vi "jrg_shellopener2.vi"() -> ()   [LabVIEW 2014]
panel:
  in  "stop":bool
  out "WaveformData":T1
  in  "Waveform index":i32
  out "Waveform Graph":waveform(dbl)(graph)
  out "error out":errorcluster
  # "MSU EFish Lab: EOD Read Display"
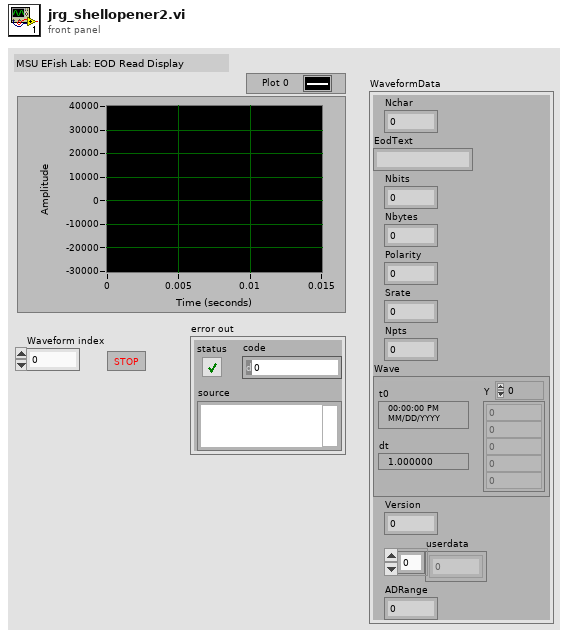
[diagram p1: front panel]
types:
  T1 = cluster{"Nchar":i32, "EodText":string, "Nbits":i32, "Nbytes":i32, "Polarity":i32, "Srate":i32, "Npts":i32, "Wave":waveform(dbl), "Version":i32, "userdata":dbl[], "ADRange":dbl}
  T2 = enum16{"open", "replace", "create", "open or create", "replace or create", "replace or create with confirmation"}
  T3 = cluster{"Nchar":i32, "EodText":string, "Nbits":i32, "Nbytes":i32, "Polarity":i32, "Srate":i32, "Npts":i32, "Wave":waveform(dbl), "Version":i32, "userdata":dbl[], "ADRange":dbl}[]
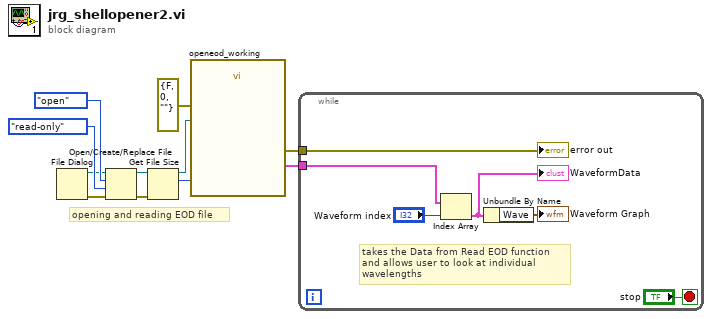
[diagram p0: block diagram]
diagram:
  # "opening and reading EOD file"
  n1 = File Dialog() -> (0:w8:errorcluster, 3:w6:path)  [unwired: 7 in, 2 out]
  n2 = Open/Create/Replace File(file path (use dialog)=w6, error in=w8, operation (0:open)=T2."open", access (0:read/write)=enum16{"read/write", "read-only", "write-only"}."read-only") -> (refnum out=w11:refnum<file>, error out=w7:errorcluster)  [unwired: 2 in, 1 out]
  n3 = Get File Size(file=w11, error in=w7) -> (refnum out=w5:refnum<file>, size (in bytes)=w4:i64)  [unwired: 1 out]
  n4 = call "openeod_working.vi"("error in (no error)"=errorcluster {"status"=FALSE, "code"=0, "source"=""}, "Byte Stream File in"=w5, "size (in bytes)"=w4) -> ("EODDataOut"=w2:T3, "error out"=w1:errorcluster)  [unwired: 14 in, 1 out]
  n5 = while {
    tunnel: w2 -> [w16]
    tunnel: w1 -> [w15]
    stop <- "stop" stop-if-true
    # "takes the Data from Read EOD function\nand allows user to look at individual\nwavelengths"
    n6 = Index Array(array=w16, index="Waveform index") -> (element=w12:T1)
    "WaveformData" <- w12
    n7 = Unbundle By Name(w12) -> ("Wave"=→"Waveform Graph":waveform(dbl))
    "error out" <- w15
  }
